vi "EnterSubroutine.vi"(8 "error in (no error)":errorcluster, 11 "AutoSubroutine in":refnum<class "AutoSubroutine.lvclass">) -> (0 "error out":errorcluster, 3 "AutoSubroutine out":refnum<class "AutoSubroutine.lvclass">)   [LabVIEW 2017, in "AutoSubroutine.lvclass"]
uses:
  AutoSubroutine.lvclass
  AutoSubroutine.lvclass/AutoSubroutine.ctl
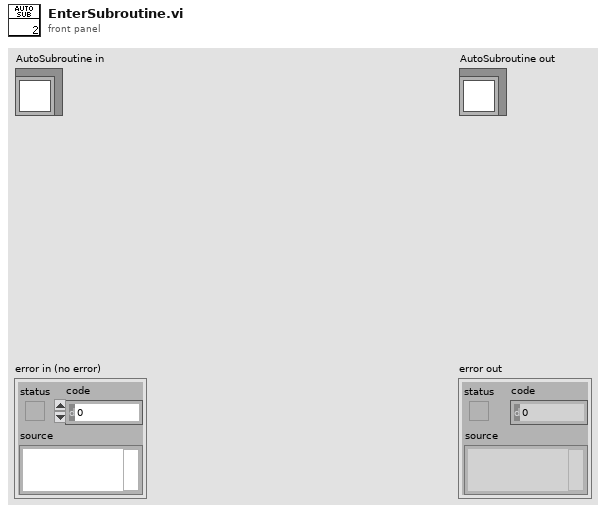
[diagram p1: front panel]
types:
  T1 = typedef "AutoSubroutine.lvclass/AutoInput.ctl" = cluster{"Start by (s)":dbl, "End by (s)":dbl, "Auto Start Time":timestamp, "Local Start":timestamp, "Okay To Start":bool, "End By Time":timestamp}
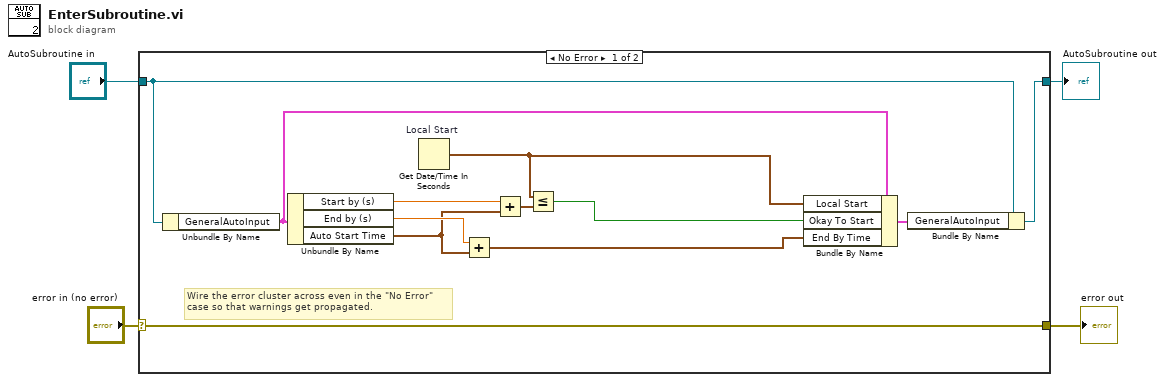
[diagram p0: block diagram]
diagram:
  n1 = case shown="No Error" "error in (no error)" {
    selector: "error in (no error)" -> [w16 w18]
    tunnel: [w16 w18] -> w3
    tunnel: [w14 w17] -> w1
    tunnel: "AutoSubroutine in" -> [w15 w17]
    frame No Error {
      # "Wire the error cluster across even in the \"No Error\"\ncase so that warnings get propagated."
      n2 = Unbundle By Name(w15) -> ("GeneralAutoInput"=w12:T1)
      n3 = Unbundle By Name(w12) -> ("Start by (s)"=w10:dbl, "End by (s)"=w9:dbl, "Auto Start Time"=w8:timestamp)
      n4 = Get Date/Time In Seconds "Local Start"() -> (seconds since 1Jan1904=w7:timestamp)
      n5 = Add(x=w9, y=w8) -> (x+y=w6:timestamp)
      n6 = Add(x=w10, y=w8) -> (x+y=w11:timestamp)
      n7 = Less Or Equal?(x=w7, y=w11) -> (x <= y?=w5:bool)
      n8 = Bundle By Name(cluster=w12, "Local Start"=w7, "Okay To Start"=w5, "End By Time"=w6) -> (w13:T1)
      n9 = Bundle By Name(cluster=w15, "GeneralAutoInput"=w13) -> (w14:refnum<class "AutoSubroutine.lvclass">)
    }
    frame Error {
    }
  }
  "error out" <- w3
  "AutoSubroutine out" <- w1
